vi "Get Build Data.vi"(8 "error in (no error)":errorcluster, 11 "NI_AB_API_Build in":refnum<class "NI_AB_API_Build.lvclass">) -> (0 "error out":errorcluster, 2 "AB_Build.lvclass":refnum<class "AB_Build.lvclass">, 3 "NI_AB_API_Build out":refnum<class "NI_AB_API_Build.lvclass">)   [LabVIEW 2020, in "NI_AB_API_Build.lvclass"]
uses:
  <vilib>/AppBuilder/AB_API/Build/NI_AB_API_Build.lvclass
  <vilib>/AppBuilder/AB_Classes/Build/AB_Build.lvclass
  <vilib>/AppBuilder/AB_API/Build/NI_AB_API_Build.lvclass/NI_AB_API_Build.ctl
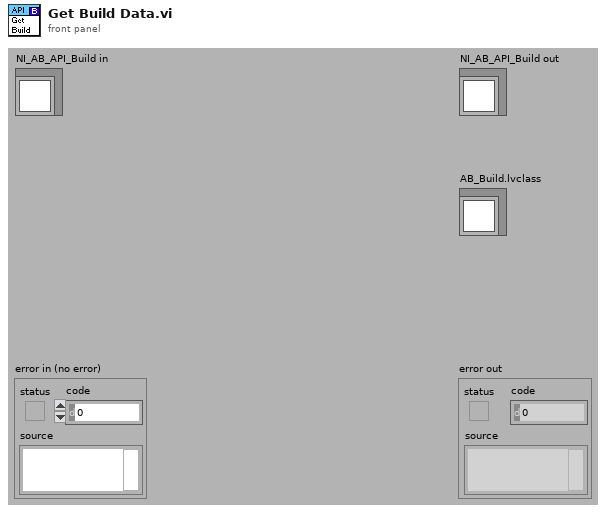
[diagram p1: front panel]
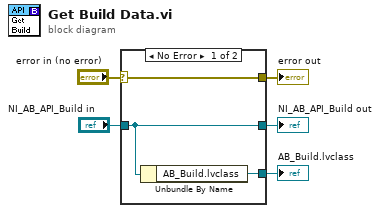
[diagram p0: block diagram]
diagram:
  n1 = case shown="No Error" "error in (no error)" {
    selector: "error in (no error)" -> [w8 w10]
    tunnel: [w8 w10] -> w4
    tunnel: [w7 w9] -> w2
    tunnel: "NI_AB_API_Build in" -> [w7 w9]
    tunnel: [w6 _] -> w1
    frame No Error {
      n2 = Unbundle By Name(w7) -> ("AB_Build.lvclass"=w6:refnum<class "AB_Build.lvclass">)
    }
    frame Error {
    }
  }
  "error out" <- w4
  "NI_AB_API_Build out" <- w2
  "AB_Build.lvclass" <- w1
